vi "Test Colour items of a string control.vi"() -> ()   [LabVIEW 2015]
uses:
  JSONtext.lvlib
panel:
  out "JSON 2":string
  in  "JSON":string
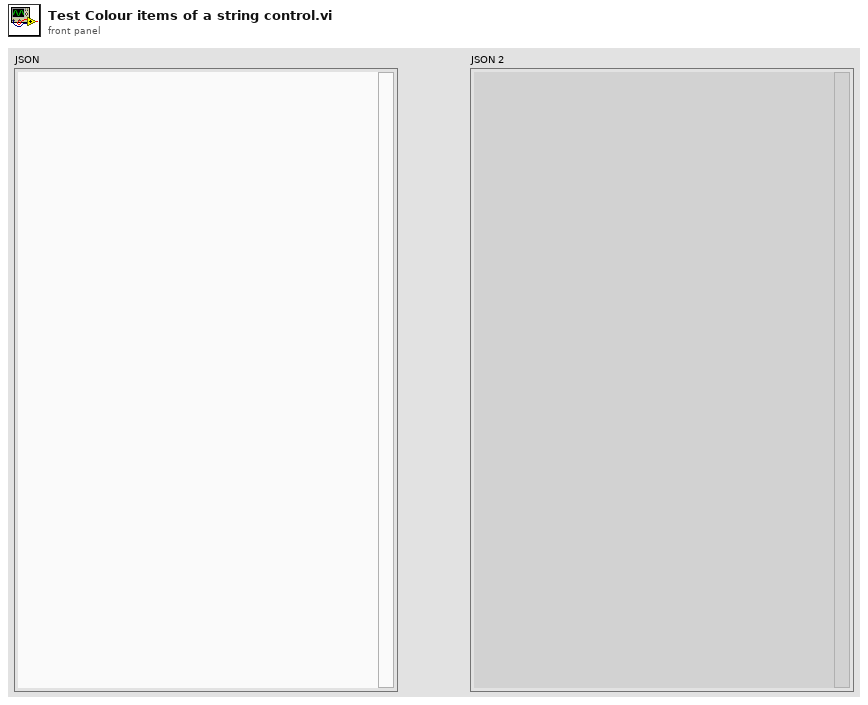
[diagram p1: front panel]
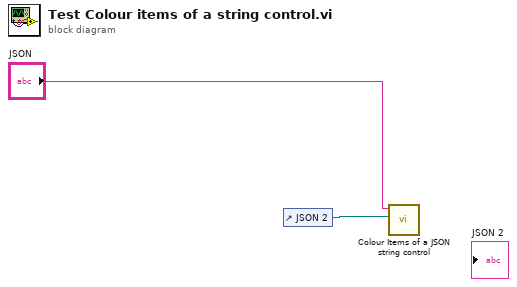
[diagram p0: block diagram]
diagram:
  n1 = control-ref of="JSON 2"() -> (w2:refnum<vi>)
  n2 = call "Colour Items of a JSON string control.vi"("String Control"=w2, "JSON"="JSON") -> ()  [unwired: 10 in]
